vi "Create User Events.vi"(8 "error in (no error)":errorcluster) -> (0 "error out":errorcluster, 3 "User Events":T1)   [LabVIEW 2018, in "User Events.lvlib"]
doc: "Create a boolean user event that will be used to stop the event loop from the message handling loop."
uses:
  User Events.lvlib
  Type Defs/User Events.ctl
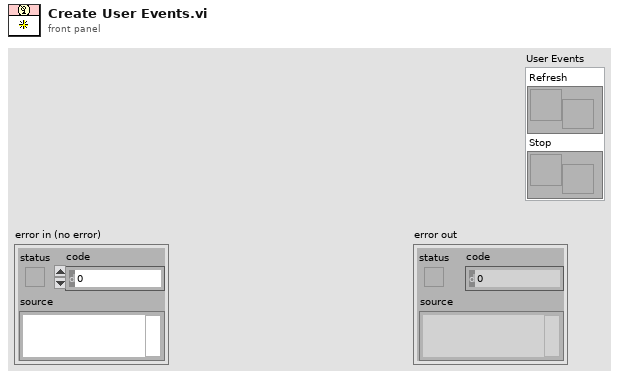
[diagram p1: front panel]
types:
  T1 = typedef "User Events.ctl" = cluster{"Refresh":refnum<user-event>, "Stop":refnum<user-event>}
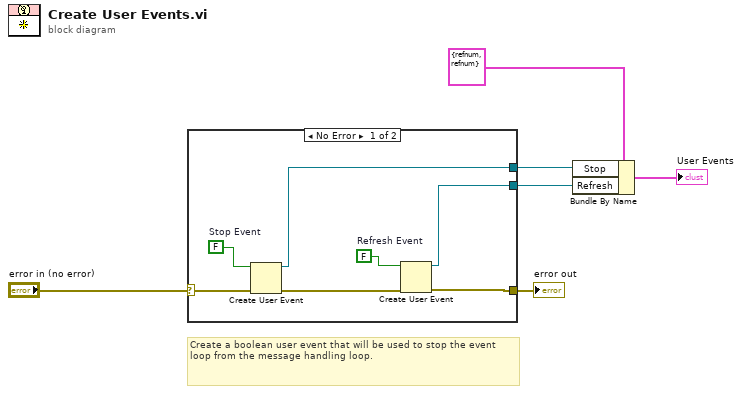
[diagram p0: block diagram]
diagram:
  # "Create a boolean user event that will be used to stop the event loop from the message handling loop."
  n1 = case shown="No Error" "error in (no error)" {
    selector: "error in (no error)" -> [w11 w14]
    tunnel: [w13 _] -> w4
    tunnel: [w9 w14] -> w6
    tunnel: [w7 _] -> w3
    frame No Error {
      w8 = FALSE  # Refresh Event
      w12 = FALSE  # Stop Event
      n2 = Create User Event(user event datatype=w12, error in=w11) -> (user event=w13:refnum<user-event>, error out=w10:errorcluster)
      n3 = Create User Event(user event datatype=w8, error in=w10) -> (user event=w7:refnum<user-event>, error out=w9:errorcluster)
    }
    frame Error {
    }
  }
  "error out" <- w6
  n4 = Bundle By Name(cluster=T1 {"Refresh"=refnum, "Stop"=refnum} ("input cluster"), "Stop"=w4, "Refresh"=w3) -> (→"User Events":T1)
